vi "addJavaScriptWithScopeElement.vi"(6 "Scope":refnum<class "tBSONDocument.lvclass">, 7 "Name":string, 8 "error in (no error)":errorcluster, 9 "Javascript":string, 10 "Replace? (false)":bool, 11 "tBSONDocument in":refnum<class "tBSONDocument.lvclass">) -> (0 "error out":errorcluster, 3 "tBSONDocument out":refnum<class "tBSONDocument.lvclass">)   [LabVIEW 2013, in "BSON.lvlib" / "tBSONDocument.lvclass"]
doc: "Adds Javascript with scope elements to a BSON document."
uses:
  tBSONDocument.lvclass
  BSONElements/tBSONJavaScriptWithScope/tBSONJavaScriptWithScope.lvclass
  tBSONElement/tBSONElement.lvclass
  tBSONElement/setName.vi
  BSONElements/tBSONJavaScript/setScript.vi
  BSONElements/tBSONJavaScriptWithScope/setScope.vi
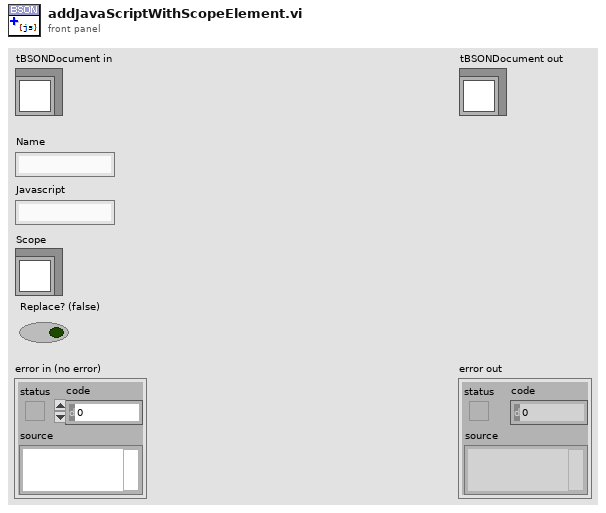
[diagram p1: front panel]
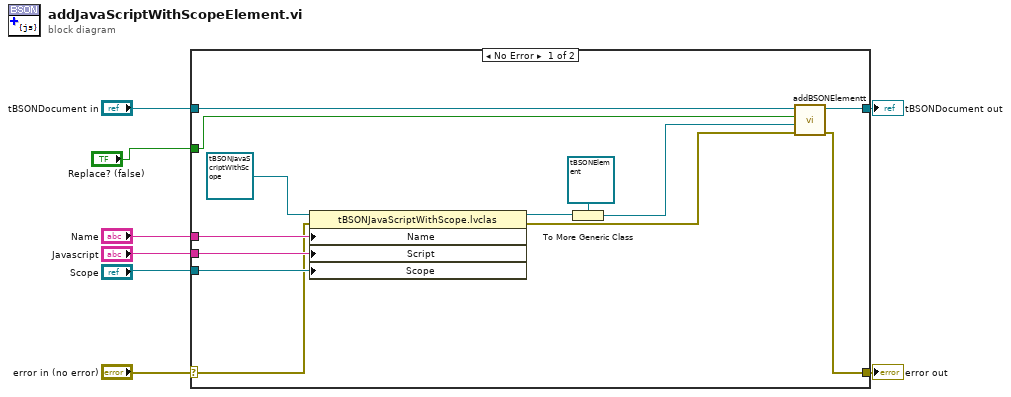
[diagram p0: block diagram]
diagram:
  n1 = case shown="No Error" "error in (no error)" {
    selector: "error in (no error)" -> [w17 w23]
    tunnel: [w12 w23] -> w7
    tunnel: [w13 w22] -> w5
    tunnel: "tBSONDocument in" -> [w14 w22]
    tunnel: "Name" -> [w20 _]
    tunnel: "Javascript" -> [w19 _]
    tunnel: "Scope" -> [w18 _]
    tunnel: "Replace? (false)" -> [w9 _]
    frame No Error {
      n2 = property class="tBSONJavaScriptWithScope.lvclas"(reference=refnum<class "tBSONJavaScriptWithScope.lvclass"> refnum ("BSON.lvlib:tBSONJavaScriptWithScope.lvclass"), error in=w17, "Name"=w20, "Script"=w19, "Scope"=w18) -> (reference out=w10:refnum<class "tBSONJavaScriptWithScope.lvclass">, error out=w11:errorcluster)
      n3 = To More Generic Class(target class=refnum<class "tBSONElement.lvclass"> refnum ("BSON.lvlib:tBSONElement.lvclass"), reference=w10) -> (generic class reference=w16:refnum<class "tBSONElement.lvclass">)
      n4 = call "addBSONElementt.vi"("error in (no error)"=w11, "Element"=w16, "Replace? (false)"=w9, "tBSONDocument in"=w14) -> ("error out"=w12:errorcluster, "tBSONDocument out"=w13:refnum<class "tBSONDocument.lvclass">)  [unwired: 6 in]
    }
    frame Error {
    }
  }
  "error out" <- w7
  "tBSONDocument out" <- w5
